vi "Write Measurements Setup.vi"(10 "Measurements Setup":T1, 11 "User Interface in":refnum<class "User Interface.lvclass">) -> (3 "User Interface out":refnum<class "User Interface.lvclass">)   [LabVIEW 2016, in "User Interface.lvlib" / "User Interface.lvclass"]
uses:
  User Interface.lvclass
  Measurements Setup.ctl
  User Interface.lvlib
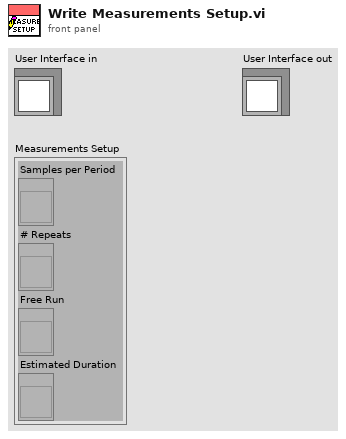
[diagram p1: front panel]
types:
  T1 = typedef "User Interface.lvlib/Measurements Setup.ctl" = cluster{"Samples per Period":refnum<vi>, "# Repeats":refnum<vi>, "Free Run":refnum<vi>, "Estimated Duration":refnum<vi>}
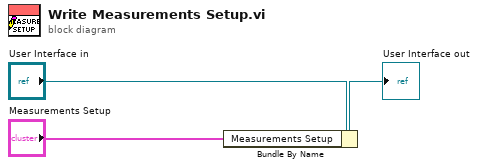
[diagram p0: block diagram]
diagram:
  n1 = Bundle By Name(cluster="User Interface in", "Measurements Setup"="Measurements Setup") -> (→"User Interface out":refnum<class "User Interface.lvclass">)
